vi "Auto_Routine_Cube_Backup_Cone.vi"(8 "error in (no error)":errorcluster) -> (0 "error out":errorcluster)   [LabVIEW 2023]
uses:
  Arm/ArmPositionPreset.ctl
  <vilib>/Rock Robotics/WPI/DriverStation/WPI_DriverStationAllianceInfo.ctl
  Arm/ArmGamePiecePreset.ctl
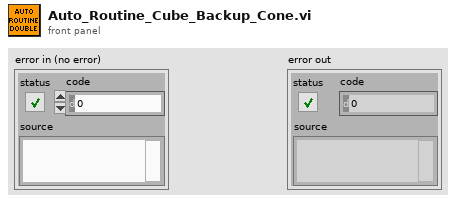
[diagram p1: front panel]
types:
  T1 = typedef "ArmGamePiecePreset.ctl" = enum16{"Cube", "Cone"}
  T2 = typedef "ArmPositionPreset.ctl" = enum16{"Upper", "Lower", "Middle", "Home", "Shelf", "Floor", "HalfFloor", "HalfHome"}
  T3 = typedef "WPI_DriverStationAllianceInfo.ctl" = enum16{"Red", "Blue", "Invalid"}
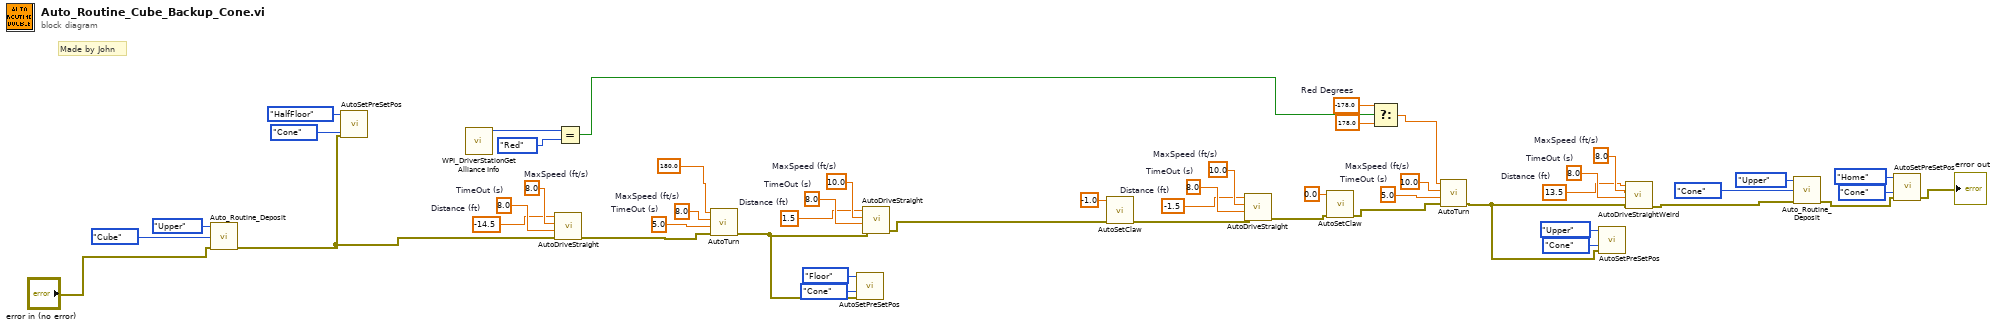
[diagram p0: block diagram]
diagram:
  w19 = -178.0  # Red Degrees
  w3 = 8.0  # TimeOut (s)
  w2 = 8.0  # MaxSpeed (ft/s)
  w1 = 13.5  # Distance (ft)
  w23 = 5.0  # TimeOut (s)
  w24 = 10.0  # MaxSpeed (ft/s)
  w28 = 8.0  # TimeOut (s)
  w29 = 10.0  # MaxSpeed (ft/s)
  w27 = -1.5  # Distance (ft)
  w31 = 8.0  # TimeOut (s)
  w32 = 10.0  # MaxSpeed (ft/s)
  w30 = 1.5  # Distance (ft)
  w36 = 5.0  # TimeOut (s)
  w37 = 8.0  # MaxSpeed (ft/s)
  w48 = 8.0  # TimeOut (s)
  w49 = 8.0  # MaxSpeed (ft/s)
  w47 = -14.5  # Distance (ft)
  # "Made by John"
  n1 = call "Auto_Routine_Deposit.vi"("error in (no error)"="error in (no error)", "Game Piece"=ArmGamePiecePreset."Cube", "Position"=ArmPositionPreset."Upper") -> ("error out"=w12:errorcluster)  [unwired: 8 in]
  n2 = call "AutoSetPreSetPos.vi"("error in (no error)"=w12, "Game Piece"=ArmGamePiecePreset."Cone", "Position"=ArmPositionPreset."HalfFloor") -> ()  [unwired: 8 in, 1 out]
  n3 = call <vilib>:"WPI_DriverStationGet Alliance Info.vi"() -> ("Alliance"=w34:T3)  [unwired: 6 in, 5 out]
  n4 = call "AutoDriveStraight.vi"("error in (no error)"=w12, "TimeOut (s)"=w48, "MaxSpeed (ft/s)"=w49, "Dist (ft)"=w47) -> ("error out"=w35:errorcluster)  [unwired: 7 in]
  n5 = Equal?(x=w34, y=WPI_DriverStationAllianceInfo."Red") -> (x = y?=w17:bool)
  n6 = call "AutoTurn.vi"("error in (no error)"=w35, "TimeOut (s)"=w36, "MaxSpeed (ft/s)"=w37, "degrees"=180.0) -> ("error out"=w11:errorcluster)  [unwired: 7 in]
  n7 = call "AutoSetPreSetPos.vi"("error in (no error)"=w11, "Game Piece"=ArmGamePiecePreset."Cone", "Position"=ArmPositionPreset."Floor") -> ()  [unwired: 8 in, 1 out]
  n8 = call "AutoDriveStraight.vi"("error in (no error)"=w11, "TimeOut (s)"=w31, "MaxSpeed (ft/s)"=w32, "Dist (ft)"=w30) -> ("error out"=w6:errorcluster)  [unwired: 7 in]
  n9 = call "AutoSetClaw.vi"("error in (no error)"=w6, "ClawDemand"=-1.0) -> ("error out"=w26:errorcluster)  [unwired: 9 in]
  n10 = call "AutoDriveStraight.vi"("error in (no error)"=w26, "TimeOut (s)"=w28, "MaxSpeed (ft/s)"=w29, "Dist (ft)"=w27) -> ("error out"=w25:errorcluster)  [unwired: 7 in]
  n11 = call "AutoSetClaw.vi"("error in (no error)"=w25, "ClawDemand"=0.0) -> ("error out"=w8:errorcluster)  [unwired: 9 in]
  n12 = Select(t=w19, s=w17, f=178.0) -> (s? t:f=w18:dbl)
  n13 = call "AutoTurn.vi"("error in (no error)"=w8, "TimeOut (s)"=w23, "MaxSpeed (ft/s)"=w24, "degrees"=w18) -> ("error out"=w4:errorcluster)  [unwired: 7 in]
  n14 = call "AutoSetPreSetPos.vi"("error in (no error)"=w4, "Game Piece"=ArmGamePiecePreset."Cone", "Position"=ArmPositionPreset."Upper") -> ()  [unwired: 8 in, 1 out]
  n15 = call "AutoDriveStraightWeird.vi"("error in (no error)"=w4, "TimeOut (s)"=w3, "MaxSpeed (ft/s)"=w2, "Dist (ft)"=w1) -> ("error out"=w5:errorcluster)  [unwired: 7 in]
  n16 = call "Auto_Routine_Deposit.vi"("error in (no error)"=w5, "Game Piece"=ArmGamePiecePreset."Cone", "Position"=ArmPositionPreset."Upper") -> ("error out"=w14:errorcluster)  [unwired: 8 in]
  n17 = call "AutoSetPreSetPos.vi"("error in (no error)"=w14, "Game Piece"=ArmGamePiecePreset."Cone", "Position"=ArmPositionPreset."Home") -> ("error out"=→"error out":errorcluster)  [unwired: 8 in]
